vi "Write Measurements.vi"(8 "error in (no error)":errorcluster, 10 "Measurements":T1, 11 "NHRDCPower in":refnum<class "NHRDCPower.lvclass">) -> (0 "error out":errorcluster, 3 "NHRDCPower out":refnum<class "NHRDCPower.lvclass">)   [LabVIEW 2018, in "AcPwrPlugins.lvlib" / "NHRDCPower.lvclass"]
uses:
  NHRDCPower.lvclass
  TypeDefs/Measurements.ctl
  NHRDCPower.lvclass/NHRDCPower.ctl
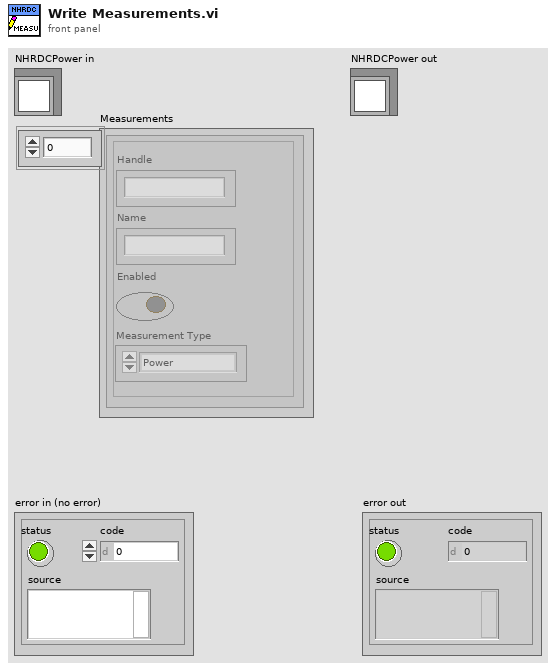
[diagram p1: front panel]
types:
  T1 = typedef "AcPwrPlugins.lvlib/NHRDCPower.lvclass/Measurements.ctl" = cluster{"Handle":string, "Name":string, "Enabled":bool, "Measurement Value":sgl, "Measurement Type":enum16{"Power", "Current", "Voltage"}}[]
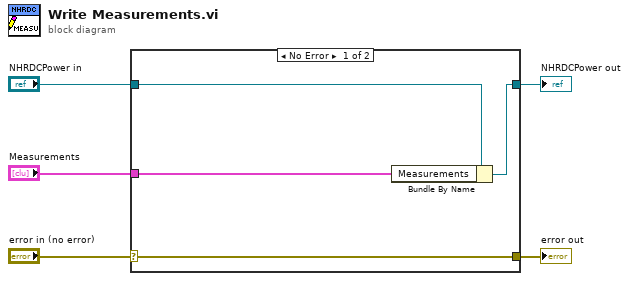
[diagram p0: block diagram]
diagram:
  n1 = case shown="No Error" "error in (no error)" {
    selector: "error in (no error)" -> [w9 w10]
    tunnel: [w9 w10] -> w4
    tunnel: [w7 w11] -> w2
    tunnel: "NHRDCPower in" -> [w8 w11]
    tunnel: "Measurements" -> [w6 _]
    frame No Error {
      n2 = Bundle By Name(cluster=w8, "Measurements"=w6) -> (w7:refnum<class "NHRDCPower.lvclass">)
    }
    frame Error {
    }
  }
  "error out" <- w4
  "NHRDCPower out" <- w2
